vi "Acquire.vi"(8 "error in (no error)":errorcluster, 11 "DAQmxDI in":refnum<class " DAQmxDI Port.lvclass">) -> (0 "error out":errorcluster, 3 "DAQmxDI out":refnum<class " DAQmxDI Port.lvclass">)   [LabVIEW 2020, in " DAQmxDI Port.lvclass"]
uses:
   DAQmxDI Port.lvclass
   DAQmxDI Port.lvclass/ DAQmxDI Port.ctl
  VolatusData/VolatusData.lvlib
  <vilib>/DAQmx/read.llb/DAQmx Read (Digital 1D Wfm NChan NSamp).vi
  <vilib>/Waveform/DWDTOps.llb/DWDT Digital to Boolean Array.vi
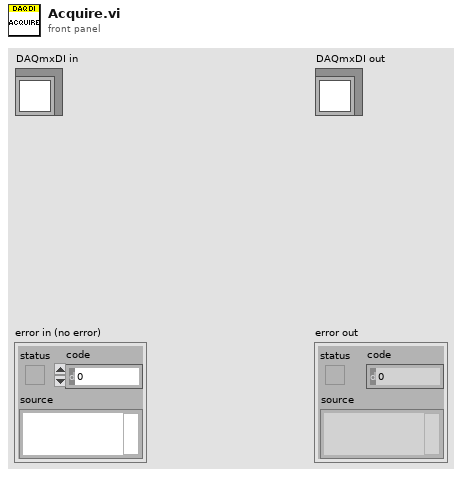
[diagram p1: front panel]
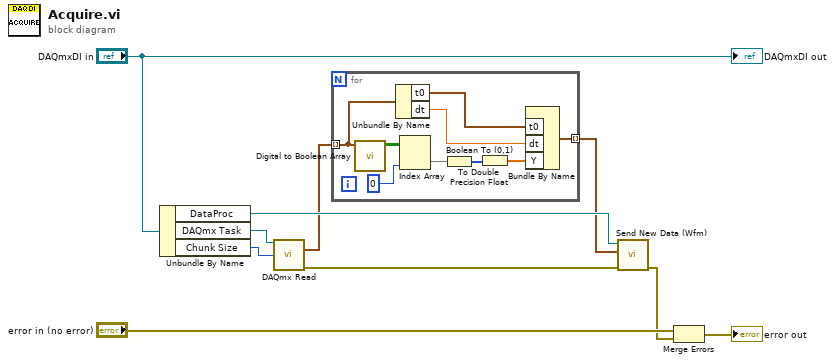
[diagram p0: block diagram]
diagram:
  n1 = Unbundle By Name("DAQmxDI in") -> ("DataProc"=w7:refnum<class "MessageQ.lvclass">, "DAQmx Task"=w9:refnum<k21>, "Chunk Size"=w8:i32)
  n2 = call-poly <vilib>:"DAQmx Read.vi"("task/channels in"=w9, "number of samples per channel"=w8) -> ("data"=w5:digitalwaveform[], "error out"=w6:errorcluster)  [unwired: 11 in, 1 out]
  n3 = for {
    tunnel: w5 -> [w16] mode=indexing
    tunnel: [w12] -> w4 mode=indexing
    n4 = call-poly <vilib>:"Digital to Boolean Array.vi"("digital waveform"=w16) -> ("boolean array"=w18:bool[][])  [unwired: 9 in, 1 out]
    n5 = Unbundle By Name(w16) -> ("t0"=w13:timestamp, "dt"=w14:dbl)
    n6 = Index Array(array=w18, index (col)=0 ("disabled index (col)")) -> (element=w17:bool[])  [unwired: 1 in]
    n7 = Boolean To (0,1)(Boolean=w17) -> (0, 1=w19:i16[])
    n8 = To Double Precision Float(number=w19) -> (double precision float=w15:dbl[])
    n9 = Bundle By Name("t0"=w13, "dt"=w14, "Y"=w15) -> (w12:waveform(dbl))  [unwired: 1 in]
  }
  n10 = call "Send New Data (Wfm).vi"("error in (no error)"=w6, "Channels"=w4, "MessageQ"=w7) -> ("error out"=w2:errorcluster)  [unwired: 8 in]
  n11 = Merge Errors("error in (no error)", w2) -> (→"error out":errorcluster)
  "DAQmxDI out" <- "DAQmxDI in"
